vi "RT Main.vi"() -> ()   [LabVIEW 2013]
uses:
  <vilib>/rvi/interface/nirviOpenFPGA/nirviOpenFPGA.xnode
  <vilib>/rvi/interface/nirviReadWriteControl/nirviReadWriteControl.xnode
  <vilib>/myRIO/Instrument Drivers/Utilities/Utilities.lvlib
  <vilib>/rvi/interface/nirviCloseFPGA/nirviCloseFPGA.xnode
  <vilib>/myRIO/Instrument Drivers/Onboard IO/DIO/DIO.lvlib
  FPGA Bitfiles/Testproj_FPGATarget_myRIO-1900Custom_x13m1FeaIu4.lvbitx
  myRIO-1900 Customized FPGA.vi
  <vilib>/FPGAPlugInAG/myRIO-1900/niLvFpga_Open_myRIO-1900.vi
  <vilib>/rvi/interface/common/dynamic/niFpgaDynamicAddResources.vi
  NiFpgaLv.dll
  <vilib>/Utility/error.llb/Error Cluster From Error Code.vi
  <vilib>/rvi/interface/Simulation/niFpgaSimulationCallBeginRW.vi
  <vilib>/rvi/errors/niLvFpgaAdjustHostInterfaceError.vi
  <vilib>/FPGAPlugInAG/Dynamic/niLvFpga_Close_Dynamic.vi
panel:
  out "Values":bool[](array[boolean])
  in  "Sonar 0":bool
  out "error out":errorcluster
  out "Acceleration":i32(graph)
  in  "Stop Button":bool
  # "Overview: The myRIO Custom FPGA Project template acquires acceleration data from the onboard accelerometer and displays the changes of acceleration values in a waveform chart. The SYS.RDY indicator shows the FPGA status.\nRequirements: LabVIEW FPGA Module.\nInstructions:\n1. Check the myRIO target IP Address in the project and make sure the target IP Address is correct. \n2. Run the VI."
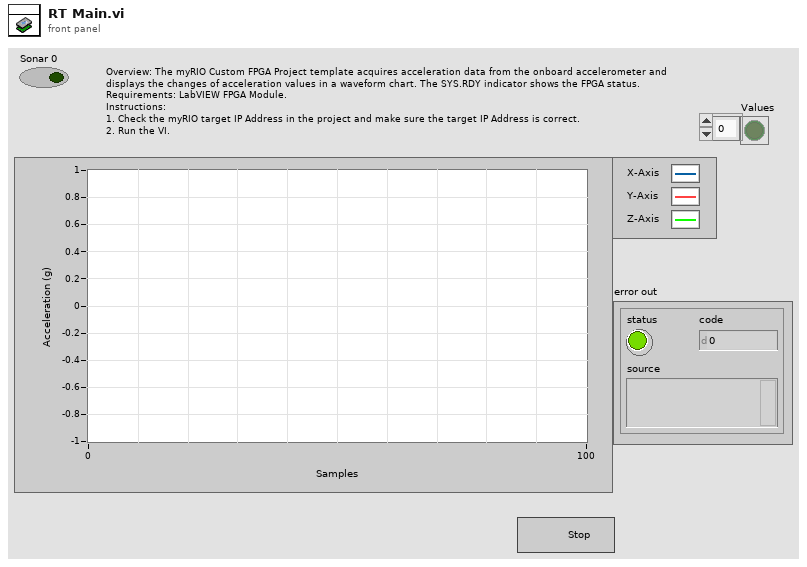
[diagram p1: front panel]
types:
  T1 = typedef "DIO.lvlib/DIO Reference.ctl" = cluster{"myRIO Reference":T2, "DIO Channels List":T6}
  T2 = typedef "myRIO Generic Hardware Reference.ctl" = cluster{"myRIO Model":T3, "myRIO Hardware Reference":T4}
  T3 = typedef "Hardware Version Enum.ctl" = enum16{"Unknown", "myRIO-1900", "myRIO-1950"}
  T4 = typedef "myRIO v1.0 Reference.ctl" = cluster{"Generic FPGA Reference":T5, "Allow multiple opens":bool}
  T5 = typedef "Generic FPGA Reference.ctl" = refnum<k20>
  T6 = typedef "DIO Channels List.ctl" = T7[]
  T7 = typedef "DIO Channels Enum.ctl" = enum16{"Not Connected", "C/DIO0", "C/DIO1", "C/DIO2", "C/DIO3", "C/DIO4", "C/DIO5", "C/DIO6", "C/DIO7", "A/DIO0", "A/DIO1", "A/DIO2", "A/DIO3", "A/DIO4", "A/DIO5", "A/DIO6", "A/DIO7", "A/DIO8", "A/DIO9", "A/DIO10", "A/DIO11", "A/DIO12", "A/DIO13", "A/DIO14", "A/DIO15", "B/DIO0", "B/DIO1", "B/DIO2", "B/DIO3", "B/DIO4", "B/DIO5", "B/DIO6", "B/DIO7", "B/DIO8", "B/DIO9", "B/DIO10", "B/DIO11", "B/DIO12", "B/DIO13", "B/DIO14", "B/DIO15", "LED0", "LED1", "LED2", "LED3", "Button0"}
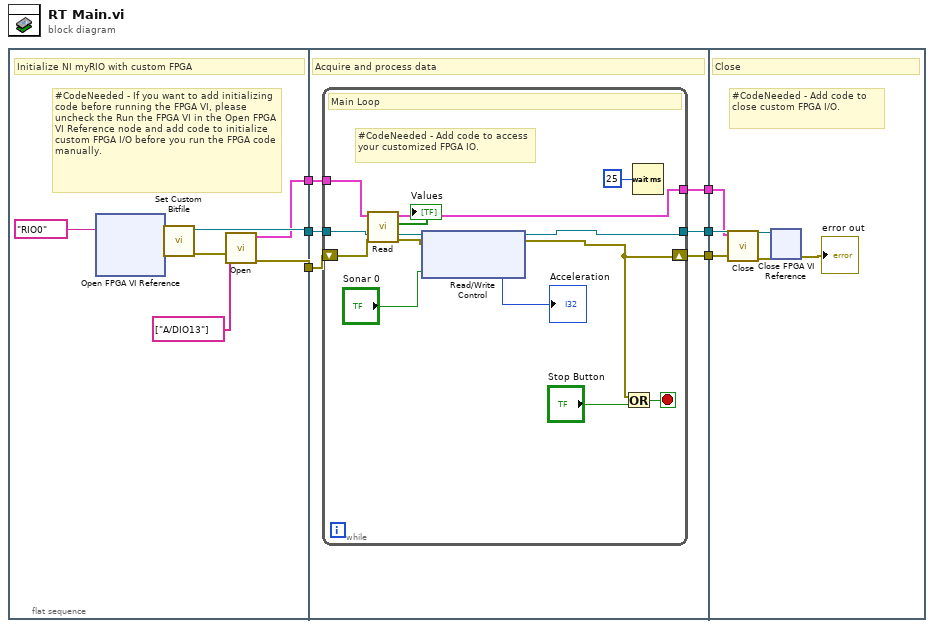
[diagram p0: block diagram]
diagram:
  n1 = flat-sequence {
    tunnel: [w11] -> w6
    tunnel: [w9] -> w3
    tunnel: [w7] -> w2
    tunnel: w6 -> [w20]
    tunnel: [w19] -> w5
    tunnel: [w18] -> w4
    tunnel: w3 -> [w17]
    tunnel: w2 -> [w16]
    tunnel: [w15] -> w1
    tunnel: w5 -> [w38]
    tunnel: w4 -> [w35]
    tunnel: w1 -> [w36]
    frame #0 {
      # "#CodeNeeded - If you want to add initializing code before running the FPGA VI, please uncheck the Run the FPGA VI in the Open FPGA VI Reference node and add code to initialize custom FPGA I/O before you run the FPGA code manually."
      # "Initialize NI myRIO with custom FPGA"
      n2 = xnode "Open FPGA VI Reference"("resource name"=tag "RIO0") -> ("FPGA VI Reference Out"=w12:refnum<k20>, "error out"=w13:errorcluster)  [unwired: 1 in]
      n3 = call <vilib>:"Set Custom Bitfile.vi"("error in (no error)"=w13, "Customized FPGA Reference in"=w12) -> ("error out"=w10:errorcluster, "Customized FPGA Reference out"=w11:refnum<k20>)  [unwired: 8 in]
      n4 = call <vilib>:"Open.vi"("error in (no error)"=w10, "Channel Names"=tag[] ["A/DIO13"]) -> ("error out"=w9:errorcluster, "DIO Ref Out"=w7:T1)  [unwired: 8 in]
    }
    frame #1 {
      # "Acquire and process data"
      n5 = while {
        tunnel: w20 -> [w31]
        tunnel: [w29] -> w19
        shift-right: [w28] -> w18
        shift-left: w17 -> [w24]
        tunnel: w16 -> [w26]
        tunnel: [w21] -> w15
        stop <- w32 stop-if-true
        # "#CodeNeeded - Add code to access your customized FPGA IO."
        # "Main Loop"
        n6 = call <vilib>:"Read.vi"("error in (no error)"=w24, "DIO Ref In"=w26) -> ("error out"=w23:errorcluster, "Values"=→"Values":bool[], "DIO Ref Out"=w21:T1)  [unwired: 7 in]
        n7 = xnode "Read/Write Control"("FPGA VI Reference In"=w31, "error in"=w23, "Sonar 0"="Sonar 0") -> ("FPGA VI Reference Out"=w29:refnum<k20>, "error out"=w28:errorcluster, "Sonar Reading 0"=→"Acceleration":i32)
        n8 = Or(x=w28, y="Stop Button") -> (x .or. y?=w32:bool)
        n9 = Wait (ms)(milliseconds to wait=u32 25) -> ()  [unwired: 1 out]
      }
    }
    frame #2 {
      # "#CodeNeeded - Add code to close custom FPGA I/O."
      # "Close"
      n10 = call <vilib>:"Close.vi"("error in (no error)"=w35, "DIO Ref In"=w36) -> ("error out"=w34:errorcluster)  [unwired: 9 in]
      n11 = xnode "Close FPGA VI Reference"("FPGA VI Reference In"=w38, "error in"=w34) -> ("error out"=→"error out":errorcluster)
    }
  }
